vi "subCalculate2TierBuildOrder.vi"(6 "UpdateList":T1, 8 "error in (no error)":errorcluster, 11 "SolutionBuilder in":refnum<class "SolutionBuilder.lvclass">) -> (0 "error out":errorcluster, 3 "SolutionBuilder out":refnum<class "SolutionBuilder.lvclass">)   [LabVIEW 2019, in "SolutionBuilder.lvlib" / "SolutionBuilder.lvclass"]
uses:
  SolutionBuilder.lvclass
  ProjectItem/ProjectItem.lvclass
  Events/EventUpdateList.ctl
  SolutionBuilder.lvlib
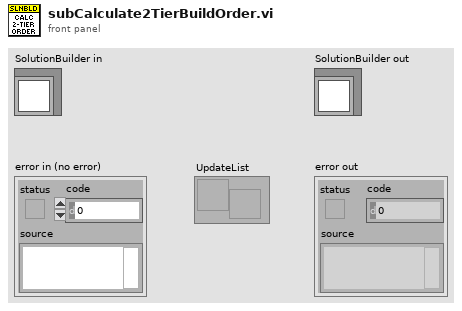
[diagram p1: front panel]
types:
  T1 = typedef "SolutionBuilder.lvlib/EventUpdateList.ctl" = refnum<user-event>
  T2 = typedef "SolutionBuilder.lvlib/SolutionBuilder.lvclass/ProjectItemMap.ctl" = map{path, refnum<class "ProjectItem.lvclass">[]}
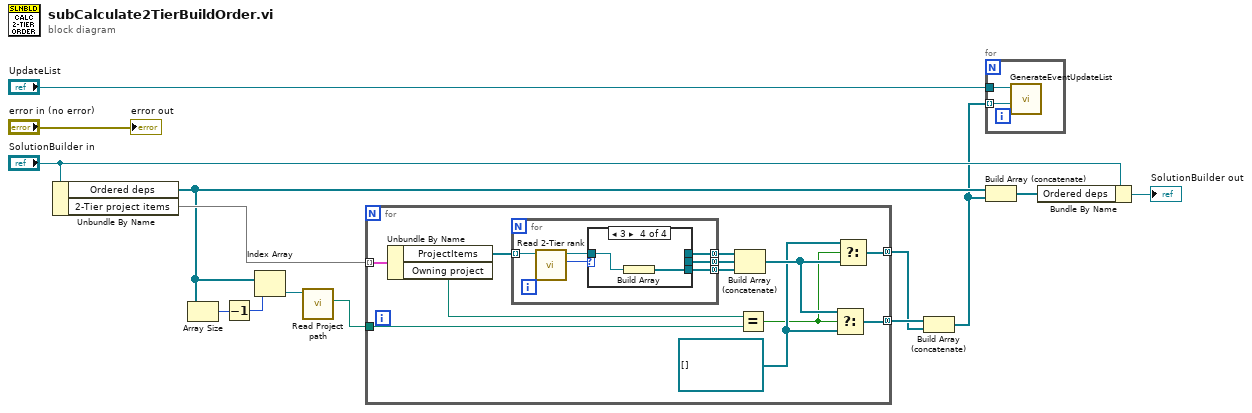
[diagram p0: block diagram]
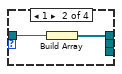
[diagram p3: hidden frame]
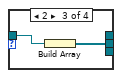
[diagram p4: hidden frame]
diagram:
  n1 = Unbundle By Name("SolutionBuilder in") -> ("Ordered deps"=w3:refnum<class "ProjectItem.lvclass">[], "2-Tier project items"=w10:T2)
  n2 = Array Size(array=w3) -> (size(s)=w13:i32)
  n3 = Decrement(x=w13) -> (x-1=w12:i32)
  n4 = Index Array(array=w3, index=w12) -> (element=w11:refnum<class "ProjectItem.lvclass">)
  n5 = call-dynamic "Read Project path.vi"("ProjectItem in"=w11) -> ("Project path"=w9:path)  [unwired: 9 in, 1 out]
  n6 = for {
    tunnel: w10 -> [w26] mode=indexing
    tunnel: w9 -> [w20]
    tunnel: [w19] -> w8 mode=concatenating
    tunnel: [w16] -> w7 mode=concatenating
    w17 = refnum<class "ProjectItem.lvclass">[] [] ("f")
    n7 = Unbundle By Name(w26) -> ("ProjectItems"=w25:refnum<class "ProjectItem.lvclass">[], "Owning project"=w21:path)
    n8 = for {
      tunnel: w25 -> [w32] mode=indexing
      tunnel: [w29] -> w24 mode=concatenating
      tunnel: [w28] -> w23 mode=concatenating
      tunnel: [w27] -> w22 mode=concatenating
      n9 = call-dynamic "Read 2-Tier rank.vi"("ProjectItem in"=w32) -> ("2-Tier rank"=w31:u8, "ProjectItem out"=w30:refnum<class "ProjectItem.lvclass">)  [unwired: 9 in]
      n10 = case shown="3" w31 {
        tunnel: w30 -> [_ w34 w36 w38]
        tunnel: [_ w33 _ _] -> w29
        tunnel: [_ _ w35 _] -> w28
        tunnel: [_ _ _ w37] -> w27
        frame 0, Default {
        }
        frame 1 {
          n11 = Build Array(w34) -> (w33:refnum<class "ProjectItem.lvclass">[])
        }
        frame 2 {
          n12 = Build Array(w36) -> (w35:refnum<class "ProjectItem.lvclass">[])
        }
        frame 3 {
          n13 = Build Array(w38) -> (w37:refnum<class "ProjectItem.lvclass">[])
        }
      }
    }
    n14 = Build Array (concatenate)(w24, w23, w22) -> (w18:refnum<class "ProjectItem.lvclass">[])
    n15 = Equal?(x=w21, y=w20) -> (x = y?=w15:bool)
    n16 = Select(t=w18, s=w15, f=w17) -> (s? t:f=w19:refnum<class "ProjectItem.lvclass">[])
    n17 = Select(t=w17, s=w15, f=w18) -> (s? t:f=w16:refnum<class "ProjectItem.lvclass">[])
  }
  n18 = Build Array (concatenate)(w8, w7) -> (w2:refnum<class "ProjectItem.lvclass">[])
  n19 = for {
    tunnel: "UpdateList" -> [w40]
    tunnel: w2 -> [w39] mode=indexing
    n20 = call "GenerateEventUpdateList.vi"("ProjectItem"=w39, "UpdateList"=w40) -> ()  [unwired: 10 in]
  }
  n21 = Build Array (concatenate)(w3, w2) -> (w1:refnum<class "ProjectItem.lvclass">[])
  n22 = Bundle By Name(cluster="SolutionBuilder in", "Ordered deps"=w1) -> (→"SolutionBuilder out":refnum<class "SolutionBuilder.lvclass">)
  "error out" <- "error in (no error)"
